vi "LAB1_ex3.vi"() -> ()   [LabVIEW 2015]
doc: "This example demonstrates how to read N channels of analog input from a LINX device."
uses:
  <vilib>/MakerHub/LINX/Public/Peripherals/Analog/Analog Read 1 Chan.vi
  <vilib>/MakerHub/LINX/Public/Peripherals/Digital/Digital Write 1 Chan.vi
  <vilib>/MakerHub/LINX/Public/Peripherals/Analog/Analog Read N Chans.vi
  <vilib>/MakerHub/LINX/Public/Peripherals/Digital/Digital Write N Chans.vi
  <vilib>/MakerHub/LINX/Private/Local IO/LinxAnalogRead.vi
  <vilib>/MakerHub/LINX/Public/Utilities/Check Channel.vi
  <vilib>/MakerHub/LINX/Private/Local IO/LinxDigitalWrite.vi
  <vilib>/MakerHub/LINX/Public/Utilities/Open Serial.vi
  <vilib>/MakerHub/LINX/Private/Utilties/Generate Error.vi
  <vilib>/MakerHub/LINX/LMH-LINX.lvlib
panel:
  in  "AI Channel":u8
  out "Analog Data":dbl(graph)
  out "Led Min":bool
  out "Led Max":bool
  in  "P_Min Threshold":dbl
  in  "P_Max Threshold":dbl
  in  "Stop Button":bool
  out "Loop Rate (Hz)":u32
  in  "Serial Port":refnum<visa-resource-name>
  # "LINX Device Settings"
  # "Analog Read N Channels Example (Serial Interface)\n\nThis example demonstrates how to read N channels of analog input values from a LINX device connected to the host computer via Serial / USB.\n\nInstructions\n1. Select the COM Port associated with the LINX Device.\n2. Select the Analog Channels to read.\n3. Click the Run Arrow."
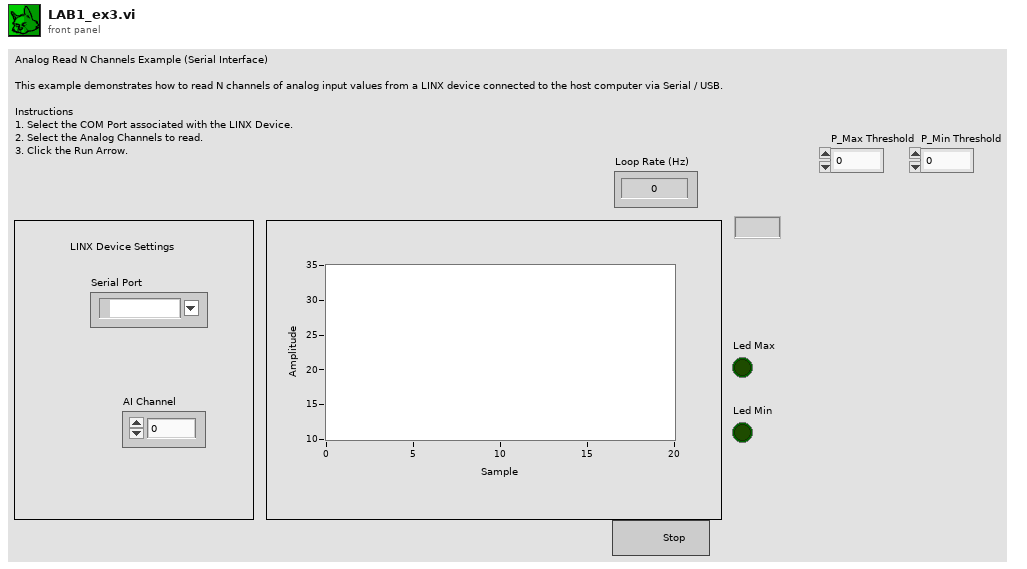
[diagram p1: front panel]
types:
  T1 = typedef "LMH-LINX.lvlib/LINX Ref.ctl" = cluster{"IO":T2, "Interface":T3, "LINX Device Config":T4}
  T2 = typedef "LMH-LINX.lvlib/Platform.ctl" = enum16{"Remote", "Local"}
  T3 = typedef "LMH-LINX.lvlib/Interface.ctl" = enum16{"Serial", "TCP"}
  T4 = typedef "LMH-LINX.lvlib/Device.lvlib/LINX Device Config.ctl" = cluster{"Interface":T3, "COM Port":refnum<visa-resource-name>, "TCP Configuration":T5, "Device Family":u8, "Device ID":u8, "Device Name":string, "TCP Ref":refnum<k5>, "Channels":T6}
  T5 = typedef "LMH-LINX.lvlib/Device.lvlib/TCP Config.ctl" = cluster{"IP Address":string, "Port":u16}
  T6 = typedef "LMH-LINX.lvlib/Channels.ctl" = cluster{"DI":u8[], "DO":u8[], "AI":u8[], "AO":u8[], "PWM":u8[], "QE":u8[], "UART":u8[], "I2C 2":u8[], "SPI":u8[], "CAN":u8[], "Servo":u8[], "AI Ref (V)":dbl, "AI Resolution (Bits)":u8, "AO Ref (V)":dbl, "AO Resolution (Bits)":u8}
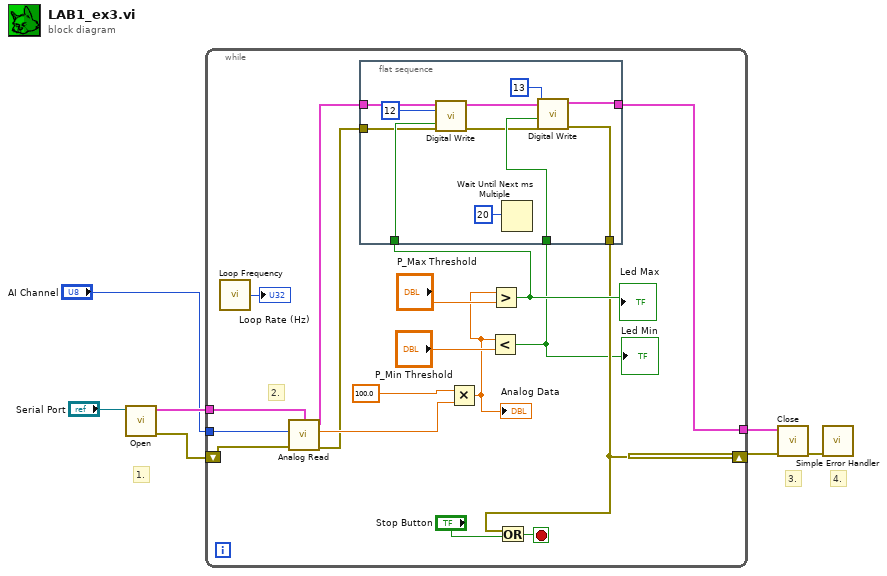
[diagram p0: block diagram]
diagram:
  # "4."
  # "3."
  # "1."
  n1 = call-poly <vilib>:"Open.vi"("Serial Port"="Serial Port") -> ("Error Out"=w6:errorcluster, "LINX Resource"=w7:T1)  [unwired: 8 in, 1 out]
  n2 = while {
    tunnel: w7 -> [w24]
    shift-right: [w11] -> w5
    shift-left: w6 -> [w23]
    tunnel: [w12] -> w2
    tunnel: "AI Channel" -> [w10]
    stop <- w22 stop-if-true
    # "2."
    n3 = call <vilib>:"Loop Frequency.vi"() -> ("Loop Rate (Hz)"=→"Loop Rate (Hz)":u32)
    n4 = call-poly <vilib>:"Analog Read.vi"("Error In"=w23, "Analog Channel"=w10, "LINX Resource"=w24) -> ("Error Out"=w13:errorcluster, "Voltage"=w16:dbl, "LINX Resource"=w14:T1)  [unwired: 5 in, 1 out]
    n5 = flat-sequence {
      tunnel: w15 -> [w34]
      tunnel: w14 -> [w31]
      tunnel: w13 -> [w33]
      tunnel: [w29] -> w12
      tunnel: w8 -> [w28]
      tunnel: [w25] -> w11
      frame #0 {
        n6 = call-poly <vilib>:"Digital Write.vi"("Error In"=w33, "Output Value"=w34, "DO Channel"=u8 12, "LINX Resource"=w31) -> ("Error Out"=w26:errorcluster, "LINX Resource"=w30:T1)  [unwired: 6 in]
        n7 = Wait Until Next ms Multiple(millisecond multiple=u32 20) -> ()  [unwired: 1 out]
        n8 = call-poly <vilib>:"Digital Write.vi"("Error In"=w26, "Output Value"=w28, "DO Channel"=u8 13, "LINX Resource"=w30) -> ("Error Out"=w25:errorcluster, "LINX Resource"=w29:T1)  [unwired: 6 in]
      }
    }
    n9 = Multiply(x=100.0, y=w16) -> (x*y=w9:dbl)
    "Analog Data" <- w9
    n10 = Less?(x=w9, y="P_Min Threshold") -> (x < y?=w8:bool)
    "Led Min" <- w8
    n11 = Greater?(x=w9, y="P_Max Threshold") -> (0:w15:bool)
    "Led Max" <- w15
    n12 = Or(x=w11, y="Stop Button") -> (x .or. y?=w22:bool)
  }
  n13 = call <vilib>:"Close.vi"("Error In"=w5, "LINX Resource"=w2) -> ("Error Out"=w3:errorcluster)  [unwired: 9 in]
  n14 = call <vilib>:"Simple Error Handler.vi"("error in (no error)"=w3) -> ()  [unwired: 4 in, 5 out]
